vi "DEC.vi"(0 "System no.":i32=1 min=1 max=4 step=1, 2 "Axes to set":string[](array[string]), 3 "Deceleration values":dbl[](array[numeric]) format="%.6f", 4 "No.of digits":i16=4, 5 "error in":errorcluster, 6 "Without axis ID?":bool) -> (14 "Controller error":bool, 19 "error out":errorcluster)   [LabVIEW 2020]
doc: "Sets closed-loop deceleration and checks for error. If Without axis ID? is TRUE, then Axes to set is ignored and first field of Deceleration values array is used for deceleration command. Number of digits is the number of digits after the decimal point in the deceleration value(s) that will be sent. Controller error is TRUE if selected system reports error code which is not 0.\n\nC-843, C-867, C-877, C-884, C-891, E-861, E-874, Mercury_GCS: Without axis ID? = FALSE. Deceleration unit is mm/s².\n\nE-873: Without axis ID? = FALSE. Deceleration unit is mm/s²."
panel:
  # "Sets closed-loop deceleration and checks for error.  If \"Without\naxis ID\" is TRUE, then \"Axes to set\" is ignored and first field of \nDeceleration values\" array is used for deceleration command."
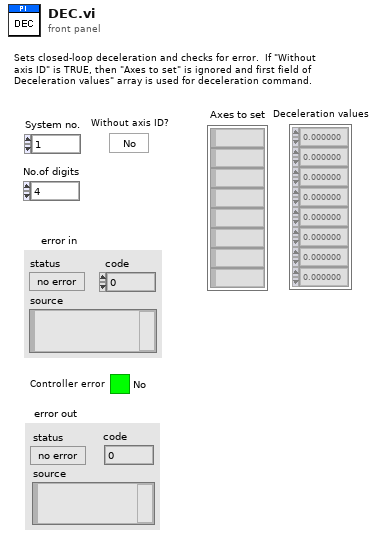
[diagram p1: front panel]
types:
  T1 = enum16{"Disable error check", "Force error check", "Use global settings"}
  T2 = typedef "Syntax.ctl" = enum16{"GCS 1.0", "GCS 2.0", "GCS 3.0"}
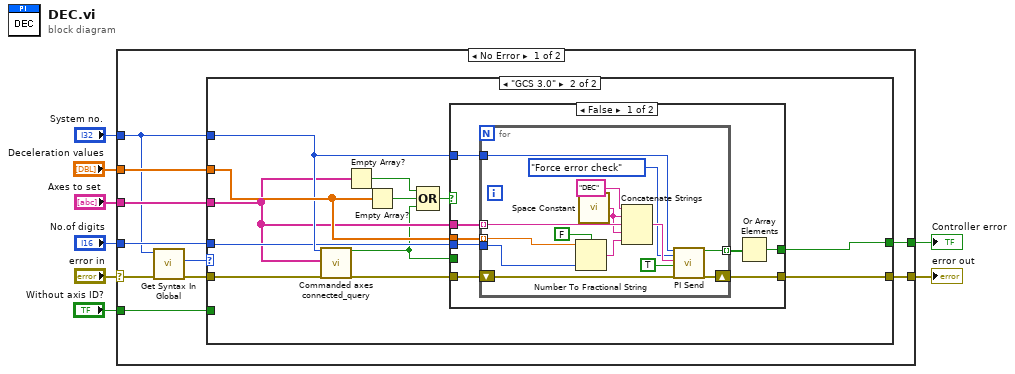
[diagram p0: block diagram]
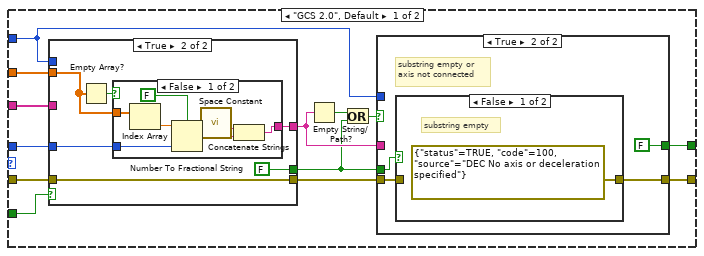
[diagram p2: hidden frame]
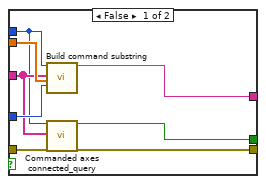
[diagram p3: hidden frame]
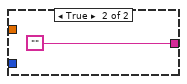
[diagram p4: hidden frame]
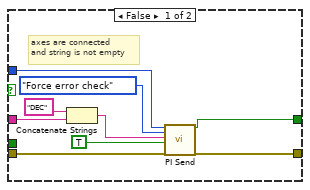
[diagram p5: hidden frame]
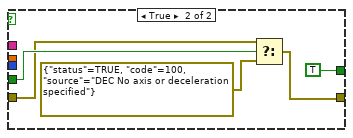
[diagram p7: hidden frame]
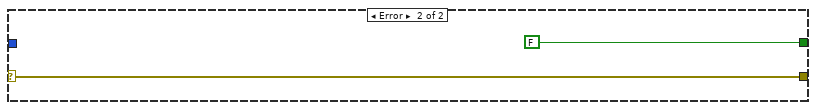
[diagram p8: hidden frame]
diagram:
  n1 = case shown="No Error" "error in" {
    selector: "error in" -> [w12 w109]
    tunnel: [w18 w109] -> w8
    tunnel: "Deceleration values" -> [w17 _]
    tunnel: "No.of digits" -> [w16 _]
    tunnel: "System no." -> [w10 _]
    tunnel: "Axes to set" -> [w15 _]
    tunnel: "Without axis ID?" -> [w14 _]
    tunnel: [w13 FALSE ("Controller error")] -> w1
    frame No Error {
      n2 = call "Get Syntax In Global.vi"("error in"=w12, "System no."=w10) -> ("error out"=w11:errorcluster, "Syntax"=w9:T2)  [unwired: 8 in]
      n3 = case shown="\"GCS 3.0\"" w9 {
        tunnel: [w31 w79] -> w18
        tunnel: w17 -> [w30 w77]
        tunnel: w16 -> [w29 w75]
        tunnel: w15 -> [w27 w74]
        tunnel: w14 -> [w25 _]
        tunnel: w10 -> [w24 w76]
        tunnel: w11 -> [w23 w78]
        tunnel: [w19 w71] -> w13
        frame "GCS 2.0", Default {
          n4 = case shown="True" w25 {
            tunnel: [w39 w43] -> w22
            tunnel: w30 -> [w38 w42]
            tunnel: w29 -> [w37 w40]
            tunnel: w23 -> [w36 w45]
            tunnel: [w35 w45] -> w28
            tunnel: w27 -> [w34 _]
            tunnel: [w33 FALSE] -> w20
            tunnel: w24 -> [w32 _]
            frame False {
              n5 = call "Build command substring.vi"("System no."=w32, "Affected axes"=w34, "Parameters"=w38, "No. of digits"=w37) -> ("Command substring"=w39:string)  [unwired: 3 in, 12 out]
              n6 = call "Commanded axes connected_query.vi"("System no."=w32, "Commanded axes"=w34, "error in"=w36) -> ("Controller error"=w33:bool, "error out"=w35:errorcluster)  [unwired: 1 in, 14 out]
            }
            frame True {
              n7 = Empty Array?(array=w42) -> (empty?=w41:bool)
              n8 = case shown="False" w41 {
                tunnel: [w51 ""] -> w43
                tunnel: w42 -> [w50 _]
                tunnel: w40 -> [w48 _]
                frame False {
                  n9 = Index Array(array=w50) -> (element=w49:dbl)  [unwired: 1 in]
                  n10 = Number To Fractional String(use system decimal point (T)=FALSE, number=w49, precision (6)=w48) -> (F-format string=w47:string)  [unwired: 1 out]
                  n11 = call "Space Constant.vi"() -> ("String"=w52:string)
                  n12 = Concatenate Strings(w52, w47) -> (w51:string)
                }
                frame True {
                }
              }
            }
          }
          n13 = Empty String/Path?(string/path=w22) -> (empty?=w21:bool)
          n14 = Or(x=w21, y=w20) -> (x .or. y?=w26:bool)
          n15 = case shown="True" w26 {
            tunnel: w22 -> [w61 _]
            tunnel: [w55 w66] -> w31
            tunnel: w28 -> [w58 w64]
            tunnel: w20 -> [_ w65]
            tunnel: w24 -> [w57 _]
            tunnel: [w56 FALSE ("Controller error")] -> w19
            frame False {
              # "axes are connected \nand string is not empty"
              n16 = Concatenate Strings("DEC", w61) -> (w59:string)
              n17 = call "PI Send.vi"("System no."=w57, "Error check settings"=T1."Force error check", "String to send"=w59, "Attach termination char.?"=TRUE ("Attach Linefeed?"), "error in"=w58) -> ("Controller error"=w56:bool, "error out"=w55:errorcluster)  [unwired: 1 in, 12 out]
            }
            frame True {
              # "substring empty or \naxis not connected"
              n18 = case shown="False" w65 {
                tunnel: [errorcluster {"status"=TRUE, "code"=100, "source"="DEC No axis or deceleration specified"} ("error out") w68] -> w66
                tunnel: w64 -> [_ w68]
                frame False {
                  # "substring empty"
                }
                frame True {
                  # "commanded axis\n not connected"
                }
              }
            }
          }
        }
        frame "GCS 3.0" {
          n19 = call "Commanded axes connected_query.vi"("System no."=w76, "Commanded axes"=w74, "error in"=w78) -> ("Controller error"=w69:bool, "error out"=w80:errorcluster)  [unwired: 15 out]
          n20 = Empty Array?(array=w74) -> (empty?=w73:bool)
          n21 = Empty Array?(array=w77) -> (empty?=w72:bool)
          n22 = Compound Arithmetic op=OR(w73, w72, w69) -> (w70:bool)
          n23 = case shown="False" w70 {
            tunnel: w80 -> [w88 w103]
            tunnel: [w87 w104] -> w79
            tunnel: w74 -> [w86 _]
            tunnel: w76 -> [w85 _]
            tunnel: w77 -> [w84 _]
            tunnel: w75 -> [w83 _]
            tunnel: [w81 TRUE] -> w71
            tunnel: w69 -> [_ w106]
            frame False {
              n24 = for {
                shift-right: [w102] -> w87
                shift-left: w88 -> [w101]
                tunnel: w86 -> [w97] mode=indexing
                tunnel: w84 -> [w94] mode=indexing
                tunnel: w85 -> [w95]
                tunnel: w83 -> [w92]
                tunnel: [w90] -> w82 mode=indexing
                n25 = Number To Fractional String(use system decimal point (T)=FALSE, number=w94, precision (6)=w92) -> (F-format string=w93:string)  [unwired: 1 in]
                n26 = call "Space Constant.vi"() -> ("String"=w96:string)
                n27 = Concatenate Strings("DEC", w96, w97, w96, w93) -> (w98:string)
                n28 = call "PI Send.vi"("System no."=w95, "Error check settings"=T1."Force error check", "String to send"=w98, "Attach termination char.?"=TRUE ("Attach Linefeed?"), "error in"=w101) -> ("Controller error"=w90:bool, "error out"=w102:errorcluster)  [unwired: 1 in, 12 out]
              }
              n29 = Or Array Elements(Boolean array=w82) -> (logical OR=w81:bool)
            }
            frame True {
              n30 = Select(t=w103, s=w106, f=errorcluster {"status"=TRUE, "code"=100, "source"="DEC No axis or deceleration specified"} ("error out")) -> (s? t:f=w104:errorcluster)
            }
          }
        }
      }
    }
    frame Error {
    }
  }
  "error out" <- w8
  "Controller error" <- w1
